vi "メイン.vi"() -> (2 "測定周期/ms":dbl, 3 "値転記用配列":T2[](array[typedef]))   [LabVIEW 2021] (continued)
                            n466 = Bundle By Name(cluster=w1247, "品質チェック項目"=w1249) -> (w1246:T2)
                          }
                          frame 7 {
                            n467 = call-poly <vilib>:"Read Key.vi"("section"=w1261, "error in (no error)"=w1260, "key"=w1257, "refnum"=w1263) -> ("error out"=w1259:errorcluster, "value"=w1258:i32, "refnum out"=w1262:T10)  [unwired: 4 in, 1 out]
                            n468 = Bundle By Name(cluster=w1256, "測定周期"=w1258) -> (w1255:T2)
                          }
                          frame 8 {
                            n469 = call-poly <vilib>:"Read Key.vi"("section"=w1270, "error in (no error)"=w1269, "key"=w1266, "refnum"=w1272) -> ("error out"=w1268:errorcluster, "value"=w1267:string, "refnum out"=w1271:T10)  [unwired: 4 in, 1 out]
                            n470 = Bundle By Name(cluster=w1264, "実測値MAX"=w1267) -> (w1265:T2)
                          }
                          frame 9 {
                            n471 = call-poly <vilib>:"Read Key.vi"("section"=w1279, "error in (no error)"=w1278, "key"=w1275, "refnum"=w1281) -> ("error out"=w1277:errorcluster, "value"=w1276:string, "refnum out"=w1280:T10)  [unwired: 4 in, 1 out]
                            n472 = Bundle By Name(cluster=w1273, "実測値MIN"=w1276) -> (w1274:T2)
                          }
                          frame 10 {
                            n473 = call-poly <vilib>:"Read Key.vi"("section"=w1288, "error in (no error)"=w1287, "key"=w1284, "refnum"=w1290) -> ("error out"=w1286:errorcluster, "value"=w1285:string, "refnum out"=w1289:T10)  [unwired: 4 in, 1 out]
                            n474 = Bundle By Name(cluster=w1282, "実測値(MAX)"=w1285) -> (w1283:T2)
                          }
                          frame 11 {
                            n475 = call-poly <vilib>:"Read Key.vi"("section"=w1297, "error in (no error)"=w1296, "key"=w1293, "refnum"=w1299) -> ("error out"=w1295:errorcluster, "value"=w1294:string, "refnum out"=w1298:T10)  [unwired: 4 in, 1 out]
                            n476 = Bundle By Name(cluster=w1291, "実測値(MIN)"=w1294) -> (w1292:T2)
                          }
                          frame 12 {
                            n477 = call-poly <vilib>:"Read Key.vi"("section"=w1306, "error in (no error)"=w1305, "key"=w1302, "refnum"=w1308) -> ("error out"=w1304:errorcluster, "value"=w1303:bool, "refnum out"=w1307:T10)  [unwired: 4 in, 1 out]
                            n478 = Bundle By Name(cluster=w1300, "測定画面表示ボタン"=w1303) -> (w1301:T2)
                          }
                          frame 13 {
                            n479 = call-poly <vilib>:"Read Key.vi"("section"=w1315, "error in (no error)"=w1314, "key"=w1311, "refnum"=w1317) -> ("error out"=w1313:errorcluster, "value"=w1312:string, "refnum out"=w1316:T10)  [unwired: 4 in, 1 out]
                            n480 = Bundle By Name(cluster=w1309, "ゲージポートNo"=w1312) -> (w1310:T2)
                          }
                        }
                        n481 = local write "メイン設定_設定 5"(w1185) -> ()
                      }
                      n482 = local read "メインON/OFF_\n設定 5"() -> (w1169:T1)
                      n483 = call-poly <vilib>:"Read Key.vi"("section"=w1158, "error in (no error)"=w1176, "key"="使用ON/OFF", "refnum"=w1177) -> ("error out"=w1161:errorcluster, "value"=w1167:bool, "refnum out"=w1162:T10)  [unwired: 4 in, 1 out]
                      n484 = Bundle By Name(cluster=w1169, "使用ON/OFF"=w1167) -> (w1170:T1)
                      n485 = local write "メインON/OFF_\n設定 5"(w1170) -> ()
                      n486 = local read "CSV項目名 5"() -> (w1165:T3)
                      n487 = call-poly <vilib>:"Read Key.vi"("section"=w1158, "error in (no error)"=w1161, "key"="CSVヘッダー名", "refnum"=w1162) -> ("error out"=w1159:errorcluster, "value"=w1163:string, "refnum out"=w1160:T10)  [unwired: 4 in, 1 out]
                      n488 = Bundle By Name(cluster=w1165, "CSV項目名"=w1163) -> (w1164:T3)
                      n489 = local write "CSV項目名 5"(w1164) -> ()
                    }
                    frame #1 {
                      # "csvヘッダー項目作成"
                      # "⑮"
                      # "⑤"
                      n490 = local read "CSV項目名 5"() -> (w1322:T3)
                      n491 = Unbundle By Name(w1322) -> ("CSV項目名"=w1319:string)
                      n492 = local read "メイン設定_設定 5"() -> (w1323:T2)
                      n493 = Unbundle By Name(w1323) -> ("測定モード"=w1318:u16)
                      n494 = case shown="0, デフォルト" w1318 {
                        tunnel: ["単発測定" _ "多点測定"] -> w1326
                        tunnel: [FALSE TRUE FALSE] -> w1325
                        tunnel: [TRUE FALSE TRUE] -> w1324
                        frame 0, Default {
                        }
                        frame 1 {
                        }
                        frame 2 {
                        }
                      }
                      n495 = case shown="1" w1318 {
                        tunnel: w1319 -> [w1332 w1344 w1353]
                        tunnel: [w1330 w1342 w1355] -> w1321
                        tunnel: [w1329 w1341 w1354] -> w1320
                        frame 1 {
                          n496 = Empty String/Path?(string/path=w1332) -> (empty?=w1331:bool)
                          n497 = case shown="FALSE" w1331 {
                            tunnel: w1332 -> [w1338 _]
                            tunnel: w1332 -> [w1337 _]
                            tunnel: [w1334 ""] -> w1330
                            tunnel: [w1333 ""] -> w1329
                            frame False {
                              n498 = Concatenate Strings(w1338, "_max") -> (w1334:string)
                              n499 = Concatenate Strings(w1337, "_min") -> (w1333:string)
                            }
                            frame True {
                            }
                          }
                        }
                        frame 2 {
                          n500 = Empty String/Path?(string/path=w1344) -> (empty?=w1343:bool)
                          n501 = case shown="FALSE" w1343 {
                            tunnel: w1344 -> [w1350 _]
                            tunnel: w1344 -> [w1349 _]
                            tunnel: [w1346 ""] -> w1342
                            tunnel: [w1345 ""] -> w1341
                            frame False {
                              n502 = Concatenate Strings(w1350, "_max") -> (w1346:string)
                              n503 = Concatenate Strings(w1349, "_min") -> (w1345:string)
                            }
                            frame True {
                            }
                          }
                        }
                        frame 0, Default {
                          n504 = Empty String/Path?(string/path=w1353) -> (empty?=w1356:bool)
                          n505 = case shown="FALSE" w1356 {
                            tunnel: w1353 -> [w1360 _]
                            tunnel: [w1358 ""] -> w1355
                            tunnel: ["" ""] -> w1354
                            frame False {
                              n506 = Concatenate Strings(w1360, "_value") -> (w1358:string)
                            }
                            frame True {
                            }
                          }
                        }
                      }
                      n507 = property on="メイン測定ボタン_単発 5" class="Bool (指定)"("BoolText.Text"=w1326) -> ()  [unwired: 2 in, 2 out]
                      n508 = local write "csv入力項目min 5"(w1320) -> ()
                      n509 = local write "csv入力項目max 5"(w1321) -> ()
                      n510 = property on="メイン測定ボタン_連続 5" class="Bool (指定)"("Visible"=w1325) -> ()  [unwired: 2 in, 2 out]
                      n511 = property on="メイン測定ボタン_単発 5" class="Bool (指定)"("Visible"=w1324) -> ()  [unwired: 2 in, 2 out]
                    }
                    frame #2 {
                      # "⑯"
                      # "⑨"
                      # "⑧"
                      # "⑦"
                      # "⑥"
                      n512 = local read "メインON/OFF_\n設定 5"() -> (w1374:T1)
                      n513 = local write "メインON/OFF_\n保存確認 5"(w1374) -> ()
                      n514 = local read "メイン設定_設定 5"() -> (w1372:T2)
                      n515 = Unbundle By Name(w1372) -> ("測定画面表示ボタン"=w1371:bool)
                      n516 = case shown="FALSE" w1371 {
                        tunnel: [w1377 TRUE] -> w1373
                        frame False {
                          w1377 = FALSE
                          n517 = property on="メイン測定ボタン_単発 5" class="Bool (指定)"("Visible"=w1377) -> ()  [unwired: 2 in, 2 out]
                          n518 = property on="メイン測定ボタン_連続 5" class="Bool (指定)"("Visible"=w1377) -> ()  [unwired: 2 in, 2 out]
                        }
                        frame True {
                        }
                      }
                      n519 = local write "メインON/OFF_制御器 5"(w1374) -> ()
                      n520 = property on="メインON/OFF_制御器 5" class="Clust (指定)"("Visible"=w1373) -> ()  [unwired: 2 in, 2 out]
                      n521 = property on="メイン設定No_設定 5" class="Clust (指定)"("Visible"=w1373) -> ()  [unwired: 2 in, 2 out]
                      n522 = property on="メイン設定_設定 5" class="Clust (指定)"("Visible"=w1373) -> ()  [unwired: 2 in, 2 out]
                      n523 = property on="キャンセルボタン 5" class="Bool (指定)"("Visible"=w1373) -> ()  [unwired: 2 in, 2 out]
                    }
                  }
                  n524 = Replace Array Subset(array=w1153, new element=w1146, index=4) -> (w1152:T2[])
                }
                frame 5 {
                  # "⑱"
                  # "⑰"
                  # "2つ目の配列に転記"
                  # "32回繰り返す為、増やす場合はこのケースストラクチャーを複製する\n複製時、設定項目の配列やボタンも複製する為、下記のボタン類の移動はしない事"
                  # "iniからデータ読み取り"
                  n525 = flat-sequence {
                    tunnel: w1388 -> [w1414]
                    tunnel: w1387 -> [w1415]
                    tunnel: [w1393] -> w1384
                    tunnel: [w1392] -> w1383
                    tunnel: w1384 -> [w1561]
                    tunnel: w1383 -> [w1560]
                    tunnel: [w1561] -> w1382
                    tunnel: [w1560] -> w1381
                    tunnel: [w1608] -> w1389
                    tunnel: [w1609] -> w1390
                    tunnel: w1382 -> [w1609]
                    tunnel: w1381 -> [w1608]
                    tunnel: [w1605] -> w1379
                    frame #0 {
                      w1391 = "設定6"
                      # "複製時に変更する項目\n①②③④⑤⑥⑦⑧⑨　⑪⑫\nローカル変数\n⑬⑭\nセレクション\n⑮⑯\nプロパティノードが\n対象配列になっているか確認\n⑰\n指標値\n⑱\n複製したケースのTrue定数を削除"
                      # "⑭"
                      # "⑬"
                      # "⑫"
                      # "⑪"
                      # "④"
                      # "③"
                      # "setting.iniファイルからの設定項目の読み取り"
                      n526 = local read "メイン設定No_設定 6"() -> (w1411:T5)
                      n527 = call-poly <vilib>:"Read Key.vi"("section"="No6.", "error in (no error)"=w1415, "key"="No.", "refnum"=w1414) -> ("error out"=w1408:errorcluster, "value"=w1412:i32, "refnum out"=w1406:T10)  [unwired: 4 in, 1 out]
                      n528 = Bundle By Name(cluster=w1411, "No."=w1412) -> (w1413:T5)
                      n529 = local write "メイン設定No_設定 6"(w1413) -> ()
                      n530 = for {
                        shift-right: [w1423] -> w1410
                        shift-left: w1406 -> [w1424]
                        shift-right: [w1420] -> w1409
                        shift-left: w1408 -> [w1421]
                        tunnel: string[] ["規格", "規格上限", "規格下限", "ポートNo.", "測定モード", "規格単位", "品質チェック項目", "測定周期", "実測MAX", "実測MIN", "実測(MAX)", "実測(MIN)", "測定画面表示ボタン", "ゲージポートNo."] -> [w1419] mode=indexing
                        tunnel: w1391 -> [w1416]
                        i -> [w1422]
                        # "②"
                        # "①"
                        n531 = local read "メイン設定_設定 6"() -> (w1417:T2)
                        n532 = case shown="0, デフォルト" w1422 {
                          tunnel: w1424 -> [w1433 w1442 w1451 w1460 w1469 w1478 w1487 w1496 w1505 w1514 w1523 w1532 w1541 w1550]
                          tunnel: [w1432 w1441 w1450 w1459 w1468 w1477 w1486 w1495 w1504 w1513 w1522 w1531 w1540 w1549] -> w1423
                          tunnel: w1416 -> [w1431 w1440 w1449 w1458 w1467 w1476 w1485 w1494 w1503 w1512 w1521 w1530 w1539 w1548]
                          tunnel: w1421 -> [w1430 w1439 w1448 w1457 w1466 w1475 w1484 w1493 w1502 w1511 w1520 w1529 w1538 w1547]
                          tunnel: [w1429 w1438 w1447 w1456 w1465 w1474 w1483 w1492 w1501 w1510 w1519 w1528 w1537 w1546] -> w1420
                          tunnel: w1419 -> [_ _ _ _ _ w1472 _ _ _ _ _ _ _ _]
                          tunnel: w1419 -> [_ _ _ _ _ _ w1481 _ _ _ _ w1526 _ _]
                          tunnel: w1419 -> [w1427 w1436 w1445 w1454 w1463 _ _ w1490 w1499 w1508 w1517 _ w1535 w1544]
                          tunnel: [w1426 w1435 w1444 w1453 w1462 w1470 w1479 w1488 w1498 w1507 w1516 w1525 w1534 w1543] -> w1418
                          tunnel: w1417 -> [w1425 w1434 w1443 w1452 w1461 w1471 w1480 w1489 w1497 w1506 w1515 w1524 w1533 w1542]
                          frame 0, Default {
                            n533 = call-poly <vilib>:"Read Key.vi"("section"=w1431, "error in (no error)"=w1430, "key"=w1427, "refnum"=w1433) -> ("error out"=w1429:errorcluster, "value"=w1428:string, "refnum out"=w1432:T10)  [unwired: 4 in, 1 out]
                            n534 = Bundle By Name(cluster=w1425, "規格"=w1428) -> (w1426:T2)
                          }
                          frame 1 {
                            n535 = call-poly <vilib>:"Read Key.vi"("section"=w1440, "error in (no error)"=w1439, "key"=w1436, "refnum"=w1442) -> ("error out"=w1438:errorcluster, "value"=w1437:string, "refnum out"=w1441:T10)  [unwired: 4 in, 1 out]
                            n536 = Bundle By Name(cluster=w1434, "規格上限"=w1437) -> (w1435:T2)
                          }
                          frame 2 {
                            n537 = call-poly <vilib>:"Read Key.vi"("section"=w1449, "error in (no error)"=w1448, "key"=w1445, "refnum"=w1451) -> ("error out"=w1447:errorcluster, "value"=w1446:string, "refnum out"=w1450:T10)  [unwired: 4 in, 1 out]
                            n538 = Bundle By Name(cluster=w1443, "規格下限"=w1446) -> (w1444:T2)
                          }
                          frame 3 {
                            n539 = call-poly <vilib>:"Read Key.vi"("section"=w1458, "error in (no error)"=w1457, "key"=w1454, "refnum"=w1460) -> ("error out"=w1456:errorcluster, "value"=w1455:i32, "refnum out"=w1459:T10)  [unwired: 4 in, 1 out]
                            n540 = Bundle By Name(cluster=w1452, "ポートNo."=w1455) -> (w1453:T2)
                          }
                          frame 4 {
                            n541 = call-poly <vilib>:"Read Key.vi"("section"=w1467, "error in (no error)"=w1466, "key"=w1463, "refnum"=w1469) -> ("error out"=w1465:errorcluster, "value"=w1464:i32, "refnum out"=w1468:T10)  [unwired: 4 in, 1 out]
                            n542 = Bundle By Name(cluster=w1461, "測定モード"=w1464) -> (w1462:T2)
                          }
                          frame 5 {
                            n543 = call-poly <vilib>:"Read Key.vi"("section"=w1476, "error in (no error)"=w1475, "key"=w1472, "refnum"=w1478) -> ("error out"=w1474:errorcluster, "value"=w1473:string, "refnum out"=w1477:T10)  [unwired: 4 in, 1 out]
                            n544 = Bundle By Name(cluster=w1471, "規格単位"=w1473) -> (w1470:T2)
                          }
                          frame 6 {
                            n545 = call-poly <vilib>:"Read Key.vi"("section"=w1485, "error in (no error)"=w1484, "key"=w1481, "refnum"=w1487) -> ("error out"=w1483:errorcluster, "value"=w1482:string, "refnum out"=w1486:T10)  [unwired: 4 in, 1 out]
                            n546 = Bundle By Name(cluster=w1480, "品質チェック項目"=w1482) -> (w1479:T2)
                          }
                          frame 7 {
                            n547 = call-poly <vilib>:"Read Key.vi"("section"=w1494, "error in (no error)"=w1493, "key"=w1490, "refnum"=w1496) -> ("error out"=w1492:errorcluster, "value"=w1491:i32, "refnum out"=w1495:T10)  [unwired: 4 in, 1 out]
                            n548 = Bundle By Name(cluster=w1489, "測定周期"=w1491) -> (w1488:T2)
                          }
                          frame 8 {
                            n549 = call-poly <vilib>:"Read Key.vi"("section"=w1503, "error in (no error)"=w1502, "key"=w1499, "refnum"=w1505) -> ("error out"=w1501:errorcluster, "value"=w1500:string, "refnum out"=w1504:T10)  [unwired: 4 in, 1 out]
                            n550 = Bundle By Name(cluster=w1497, "実測値MAX"=w1500) -> (w1498:T2)
                          }
                          frame 9 {
                            n551 = call-poly <vilib>:"Read Key.vi"("section"=w1512, "error in (no error)"=w1511, "key"=w1508, "refnum"=w1514) -> ("error out"=w1510:errorcluster, "value"=w1509:string, "refnum out"=w1513:T10)  [unwired: 4 in, 1 out]
                            n552 = Bundle By Name(cluster=w1506, "実測値MIN"=w1509) -> (w1507:T2)
                          }
                          frame 10 {
                            n553 = call-poly <vilib>:"Read Key.vi"("section"=w1521, "error in (no error)"=w1520, "key"=w1517, "refnum"=w1523) -> ("error out"=w1519:errorcluster, "value"=w1518:string, "refnum out"=w1522:T10)  [unwired: 4 in, 1 out]
                            n554 = Bundle By Name(cluster=w1515, "実測値(MAX)"=w1518) -> (w1516:T2)
                          }
                          frame 11 {
                            n555 = call-poly <vilib>:"Read Key.vi"("section"=w1530, "error in (no error)"=w1529, "key"=w1526, "refnum"=w1532) -> ("error out"=w1528:errorcluster, "value"=w1527:string, "refnum out"=w1531:T10)  [unwired: 4 in, 1 out]
                            n556 = Bundle By Name(cluster=w1524, "実測値(MIN)"=w1527) -> (w1525:T2)
                          }
                          frame 12 {
                            n557 = call-poly <vilib>:"Read Key.vi"("section"=w1539, "error in (no error)"=w1538, "key"=w1535, "refnum"=w1541) -> ("error out"=w1537:errorcluster, "value"=w1536:bool, "refnum out"=w1540:T10)  [unwired: 4 in, 1 out]
                            n558 = Bundle By Name(cluster=w1533, "測定画面表示ボタン"=w1536) -> (w1534:T2)
                          }
                          frame 13 {
                            n559 = call-poly <vilib>:"Read Key.vi"("section"=w1548, "error in (no error)"=w1547, "key"=w1544, "refnum"=w1550) -> ("error out"=w1546:errorcluster, "value"=w1545:string, "refnum out"=w1549:T10)  [unwired: 4 in, 1 out]
                            n560 = Bundle By Name(cluster=w1542, "ゲージポートNo"=w1545) -> (w1543:T2)
                          }
                        }
                        n561 = local write "メイン設定_設定 6"(w1418) -> ()
                      }
                      n562 = local read "メインON/OFF_\n設定 6"() -> (w1402:T1)
                      n563 = call-poly <vilib>:"Read Key.vi"("section"=w1391, "error in (no error)"=w1409, "key"="使用ON/OFF", "refnum"=w1410) -> ("error out"=w1394:errorcluster, "value"=w1400:bool, "refnum out"=w1395:T10)  [unwired: 4 in, 1 out]
                      n564 = Bundle By Name(cluster=w1402, "使用ON/OFF"=w1400) -> (w1403:T1)
                      n565 = local write "メインON/OFF_\n設定 6"(w1403) -> ()
                      n566 = local read "CSV項目名 6"() -> (w1398:T3)
                      n567 = call-poly <vilib>:"Read Key.vi"("section"=w1391, "error in (no error)"=w1394, "key"="CSVヘッダー名", "refnum"=w1395) -> ("error out"=w1392:errorcluster, "value"=w1396:string, "refnum out"=w1393:T10)  [unwired: 4 in, 1 out]
                      n568 = Bundle By Name(cluster=w1398, "CSV項目名"=w1396) -> (w1397:T3)
                      n569 = local write "CSV項目名 6"(w1397) -> ()
                    }
                    frame #1 {
                      # "csvヘッダー項目作成"
                      # "⑮"
                      # "⑤"
                      n570 = local read "CSV項目名 6"() -> (w1555:T3)
                      n571 = Unbundle By Name(w1555) -> ("CSV項目名"=w1552:string)
                      n572 = local read "メイン設定_設定 6"() -> (w1556:T2)
                      n573 = Unbundle By Name(w1556) -> ("測定モード"=w1551:u16)
                      n574 = case shown="0, デフォルト" w1551 {
                        tunnel: ["単発測定" _ "多点測定"] -> w1559
                        tunnel: [FALSE TRUE FALSE] -> w1558
                        tunnel: [TRUE FALSE TRUE] -> w1557
                        frame 0, Default {
                        }
                        frame 1 {
                        }
                        frame 2 {
                        }
                      }
                      n575 = case shown="1" w1551 {
                        tunnel: w1552 -> [w1565 w1577 w1586]
                        tunnel: [w1563 w1575 w1588] -> w1554
                        tunnel: [w1562 w1574 w1587] -> w1553
                        frame 1 {
                          n576 = Empty String/Path?(string/path=w1565) -> (empty?=w1564:bool)
                          n577 = case shown="FALSE" w1564 {
                            tunnel: w1565 -> [w1571 _]
                            tunnel: w1565 -> [w1570 _]
                            tunnel: [w1567 ""] -> w1563
                            tunnel: [w1566 ""] -> w1562
                            frame False {
                              n578 = Concatenate Strings(w1571, "_max") -> (w1567:string)
                              n579 = Concatenate Strings(w1570, "_min") -> (w1566:string)
                            }
                            frame True {
                            }
                          }
                        }
                        frame 2 {
                          n580 = Empty String/Path?(string/path=w1577) -> (empty?=w1576:bool)
                          n581 = case shown="FALSE" w1576 {
                            tunnel: w1577 -> [w1583 _]
                            tunnel: w1577 -> [w1582 _]
                            tunnel: [w1579 ""] -> w1575
                            tunnel: [w1578 ""] -> w1574
                            frame False {
                              n582 = Concatenate Strings(w1583, "_max") -> (w1579:string)
                              n583 = Concatenate Strings(w1582, "_min") -> (w1578:string)
                            }
                            frame True {
                            }
                          }
                        }
                        frame 0, Default {
                          n584 = Empty String/Path?(string/path=w1586) -> (empty?=w1589:bool)
                          n585 = case shown="FALSE" w1589 {
                            tunnel: w1586 -> [w1593 _]
                            tunnel: [w1591 ""] -> w1588
                            tunnel: ["" ""] -> w1587
                            frame False {
                              n586 = Concatenate Strings(w1593, "_value") -> (w1591:string)
                            }
                            frame True {
                            }
                          }
                        }
                      }
                      n587 = property on="メイン測定ボタン_単発 6" class="Bool (指定)"("BoolText.Text"=w1559) -> ()  [unwired: 2 in, 2 out]
                      n588 = local write "csv入力項目min 6"(w1553) -> ()
                      n589 = local write "csv入力項目max 6"(w1554) -> ()
                      n590 = property on="メイン測定ボタン_連続 6" class="Bool (指定)"("Visible"=w1558) -> ()  [unwired: 2 in, 2 out]
                      n591 = property on="メイン測定ボタン_単発 6" class="Bool (指定)"("Visible"=w1557) -> ()  [unwired: 2 in, 2 out]
                    }
                    frame #2 {
                      # "⑯"
                      # "⑨"
                      # "⑧"
                      # "⑦"
                      # "⑥"
                      n592 = local read "メインON/OFF_\n設定 6"() -> (w1607:T1)
                      n593 = local write "メインON/OFF_\n保存確認 6"(w1607) -> ()
                      n594 = local read "メイン設定_設定 6"() -> (w1605:T2)
                      n595 = Unbundle By Name(w1605) -> ("測定画面表示ボタン"=w1604:bool)
                      n596 = case shown="FALSE" w1604 {
                        tunnel: [w1610 TRUE] -> w1606
                        frame False {
                          w1610 = FALSE
                          n597 = property on="メイン測定ボタン_単発 6" class="Bool (指定)"("Visible"=w1610) -> ()  [unwired: 2 in, 2 out]
                          n598 = property on="メイン測定ボタン_連続 6" class="Bool (指定)"("Visible"=w1610) -> ()  [unwired: 2 in, 2 out]
                        }
                        frame True {
                        }
                      }
                      n599 = local write "メインON/OFF_制御器 6"(w1607) -> ()
                      n600 = property on="メインON/OFF_制御器 6" class="Clust (指定)"("Visible"=w1606) -> ()  [unwired: 2 in, 2 out]
                      n601 = property on="メイン設定No_設定 6" class="Clust (指定)"("Visible"=w1606) -> ()  [unwired: 2 in, 2 out]
                      n602 = property on="メイン設定_設定 6" class="Clust (指定)"("Visible"=w1606) -> ()  [unwired: 2 in, 2 out]
                      n603 = property on="キャンセルボタン 6" class="Bool (指定)"("Visible"=w1606) -> ()  [unwired: 2 in, 2 out]
                    }
                  }
                  n604 = Replace Array Subset(array=w1386, new element=w1379, index=5) -> (w1385:T2[])
                }
                frame 6 {
                  # "⑱"
                  # "⑰"
                  # "2つ目の配列に転記"
                  # "32回繰り返す為、増やす場合はこのケースストラクチャーを複製する\n複製時、設定項目の配列やボタンも複製する為、下記のボタン類の移動はしない事"
                  # "iniからデータ読み取り"
                  n605 = flat-sequence {
                    tunnel: w1621 -> [w1647]
                    tunnel: w1620 -> [w1648]
                    tunnel: [w1626] -> w1617
                    tunnel: [w1625] -> w1616
                    tunnel: w1617 -> [w1794]
                    tunnel: w1616 -> [w1793]
                    tunnel: [w1794] -> w1615
                    tunnel: [w1793] -> w1614
                    tunnel: [w1841] -> w1622
                    tunnel: [w1842] -> w1623
                    tunnel: w1615 -> [w1842]
                    tunnel: w1614 -> [w1841]
                    tunnel: [w1838] -> w1612
                    frame #0 {
                      w1624 = "設定7"
                      # "複製時に変更する項目\n①②③④⑤⑥⑦⑧⑨　⑪⑫\nローカル変数\n⑬⑭\nセレクション\n⑮⑯\nプロパティノードが\n対象配列になっているか確認\n⑰\n指標値\n⑱\n複製したケースのTrue定数を削除"
                      # "⑭"
                      # "⑬"
                      # "⑫"
                      # "⑪"
                      # "④"
                      # "③"
                      # "setting.iniファイルからの設定項目の読み取り"
                      n606 = local read "メイン設定No_設定 7"() -> (w1644:T5)
                      n607 = call-poly <vilib>:"Read Key.vi"("section"="No7.", "error in (no error)"=w1648, "key"="No.", "refnum"=w1647) -> ("error out"=w1641:errorcluster, "value"=w1645:i32, "refnum out"=w1639:T10)  [unwired: 4 in, 1 out]
                      n608 = Bundle By Name(cluster=w1644, "No."=w1645) -> (w1646:T5)
                      n609 = local write "メイン設定No_設定 7"(w1646) -> ()
                      n610 = for {
                        shift-right: [w1656] -> w1643
                        shift-left: w1639 -> [w1657]
                        shift-right: [w1653] -> w1642
                        shift-left: w1641 -> [w1654]
                        tunnel: string[] ["規格", "規格上限", "規格下限", "ポートNo.", "測定モード", "規格単位", "品質チェック項目", "測定周期", "実測MAX", "実測MIN", "実測(MAX)", "実測(MIN)", "測定画面表示ボタン", "ゲージポートNo."] -> [w1652] mode=indexing
                        tunnel: w1624 -> [w1649]
                        i -> [w1655]
                        # "②"
                        # "①"
                        n611 = local read "メイン設定_設定 7"() -> (w1650:T2)
                        n612 = case shown="0, デフォルト" w1655 {
                          tunnel: w1657 -> [w1666 w1675 w1684 w1693 w1702 w1711 w1720 w1729 w1738 w1747 w1756 w1765 w1774 w1783]
                          tunnel: [w1665 w1674 w1683 w1692 w1701 w1710 w1719 w1728 w1737 w1746 w1755 w1764 w1773 w1782] -> w1656
                          tunnel: w1649 -> [w1664 w1673 w1682 w1691 w1700 w1709 w1718 w1727 w1736 w1745 w1754 w1763 w1772 w1781]
                          tunnel: w1654 -> [w1663 w1672 w1681 w1690 w1699 w1708 w1717 w1726 w1735 w1744 w1753 w1762 w1771 w1780]
                          tunnel: [w1662 w1671 w1680 w1689 w1698 w1707 w1716 w1725 w1734 w1743 w1752 w1761 w1770 w1779] -> w1653
                          tunnel: w1652 -> [_ _ _ _ _ w1705 _ _ _ _ _ _ _ _]
                          tunnel: w1652 -> [_ _ _ _ _ _ w1714 _ _ _ _ w1759 _ _]
                          tunnel: w1652 -> [w1660 w1669 w1678 w1687 w1696 _ _ w1723 w1732 w1741 w1750 _ w1768 w1777]
                          tunnel: [w1659 w1668 w1677 w1686 w1695 w1703 w1712 w1721 w1731 w1740 w1749 w1758 w1767 w1776] -> w1651
                          tunnel: w1650 -> [w1658 w1667 w1676 w1685 w1694 w1704 w1713 w1722 w1730 w1739 w1748 w1757 w1766 w1775]
                          frame 0, Default {
                            n613 = call-poly <vilib>:"Read Key.vi"("section"=w1664, "error in (no error)"=w1663, "key"=w1660, "refnum"=w1666) -> ("error out"=w1662:errorcluster, "value"=w1661:string, "refnum out"=w1665:T10)  [unwired: 4 in, 1 out]
                            n614 = Bundle By Name(cluster=w1658, "規格"=w1661) -> (w1659:T2)
                          }
                          frame 1 {
                            n615 = call-poly <vilib>:"Read Key.vi"("section"=w1673, "error in (no error)"=w1672, "key"=w1669, "refnum"=w1675) -> ("error out"=w1671:errorcluster, "value"=w1670:string, "refnum out"=w1674:T10)  [unwired: 4 in, 1 out]
                            n616 = Bundle By Name(cluster=w1667, "規格上限"=w1670) -> (w1668:T2)
                          }
                          frame 2 {
                            n617 = call-poly <vilib>:"Read Key.vi"("section"=w1682, "error in (no error)"=w1681, "key"=w1678, "refnum"=w1684) -> ("error out"=w1680:errorcluster, "value"=w1679:string, "refnum out"=w1683:T10)  [unwired: 4 in, 1 out]
                            n618 = Bundle By Name(cluster=w1676, "規格下限"=w1679) -> (w1677:T2)
                          }
                          frame 3 {
                            n619 = call-poly <vilib>:"Read Key.vi"("section"=w1691, "error in (no error)"=w1690, "key"=w1687, "refnum"=w1693) -> ("error out"=w1689:errorcluster, "value"=w1688:i32, "refnum out"=w1692:T10)  [unwired: 4 in, 1 out]
                            n620 = Bundle By Name(cluster=w1685, "ポートNo."=w1688) -> (w1686:T2)
                          }
                          frame 4 {
                            n621 = call-poly <vilib>:"Read Key.vi"("section"=w1700, "error in (no error)"=w1699, "key"=w1696, "refnum"=w1702) -> ("error out"=w1698:errorcluster, "value"=w1697:i32, "refnum out"=w1701:T10)  [unwired: 4 in, 1 out]
                            n622 = Bundle By Name(cluster=w1694, "測定モード"=w1697) -> (w1695:T2)
                          }
                          frame 5 {
                            n623 = call-poly <vilib>:"Read Key.vi"("section"=w1709, "error in (no error)"=w1708, "key"=w1705, "refnum"=w1711) -> ("error out"=w1707:errorcluster, "value"=w1706:string, "refnum out"=w1710:T10)  [unwired: 4 in, 1 out]
                            n624 = Bundle By Name(cluster=w1704, "規格単位"=w1706) -> (w1703:T2)
                          }
                          frame 6 {
                            n625 = call-poly <vilib>:"Read Key.vi"("section"=w1718, "error in (no error)"=w1717, "key"=w1714, "refnum"=w1720) -> ("error out"=w1716:errorcluster, "value"=w1715:string, "refnum out"=w1719:T10)  [unwired: 4 in, 1 out]
                            n626 = Bundle By Name(cluster=w1713, "品質チェック項目"=w1715) -> (w1712:T2)
                          }
                          frame 7 {
                            n627 = call-poly <vilib>:"Read Key.vi"("section"=w1727, "error in (no error)"=w1726, "key"=w1723, "refnum"=w1729) -> ("error out"=w1725:errorcluster, "value"=w1724:i32, "refnum out"=w1728:T10)  [unwired: 4 in, 1 out]
                            n628 = Bundle By Name(cluster=w1722, "測定周期"=w1724) -> (w1721:T2)
                          }
                          frame 8 {
                            n629 = call-poly <vilib>:"Read Key.vi"("section"=w1736, "error in (no error)"=w1735, "key"=w1732, "refnum"=w1738) -> ("error out"=w1734:errorcluster, "value"=w1733:string, "refnum out"=w1737:T10)  [unwired: 4 in, 1 out]
                            n630 = Bundle By Name(cluster=w1730, "実測値MAX"=w1733) -> (w1731:T2)
                          }
                          frame 9 {
                            n631 = call-poly <vilib>:"Read Key.vi"("section"=w1745, "error in (no error)"=w1744, "key"=w1741, "refnum"=w1747) -> ("error out"=w1743:errorcluster, "value"=w1742:string, "refnum out"=w1746:T10)  [unwired: 4 in, 1 out]
                            n632 = Bundle By Name(cluster=w1739, "実測値MIN"=w1742) -> (w1740:T2)
                          }
                          frame 10 {
                            n633 = call-poly <vilib>:"Read Key.vi"("section"=w1754, "error in (no error)"=w1753, "key"=w1750, "refnum"=w1756) -> ("error out"=w1752:errorcluster, "value"=w1751:string, "refnum out"=w1755:T10)  [unwired: 4 in, 1 out]
                            n634 = Bundle By Name(cluster=w1748, "実測値(MAX)"=w1751) -> (w1749:T2)
                          }
                          frame 11 {
                            n635 = call-poly <vilib>:"Read Key.vi"("section"=w1763, "error in (no error)"=w1762, "key"=w1759, "refnum"=w1765) -> ("error out"=w1761:errorcluster, "value"=w1760:string, "refnum out"=w1764:T10)  [unwired: 4 in, 1 out]
                            n636 = Bundle By Name(cluster=w1757, "実測値(MIN)"=w1760) -> (w1758:T2)
                          }
                          frame 12 {
                            n637 = call-poly <vilib>:"Read Key.vi"("section"=w1772, "error in (no error)"=w1771, "key"=w1768, "refnum"=w1774) -> ("error out"=w1770:errorcluster, "value"=w1769:bool, "refnum out"=w1773:T10)  [unwired: 4 in, 1 out]
                            n638 = Bundle By Name(cluster=w1766, "測定画面表示ボタン"=w1769) -> (w1767:T2)
                          }
                          frame 13 {
                            n639 = call-poly <vilib>:"Read Key.vi"("section"=w1781, "error in (no error)"=w1780, "key"=w1777, "refnum"=w1783) -> ("error out"=w1779:errorcluster, "value"=w1778:string, "refnum out"=w1782:T10)  [unwired: 4 in, 1 out]
                            n640 = Bundle By Name(cluster=w1775, "ゲージポートNo"=w1778) -> (w1776:T2)
                          }
                        }
                        n641 = local write "メイン設定_設定 7"(w1651) -> ()
                      }
                      n642 = local read "メインON/OFF_\n設定 7"() -> (w1635:T1)
                      n643 = call-poly <vilib>:"Read Key.vi"("section"=w1624, "error in (no error)"=w1642, "key"="使用ON/OFF", "refnum"=w1643) -> ("error out"=w1627:errorcluster, "value"=w1633:bool, "refnum out"=w1628:T10)  [unwired: 4 in, 1 out]
                      n644 = Bundle By Name(cluster=w1635, "使用ON/OFF"=w1633) -> (w1636:T1)
                      n645 = local write "メインON/OFF_\n設定 7"(w1636) -> ()
                      n646 = local read "CSV項目名 7"() -> (w1631:T3)
                      n647 = call-poly <vilib>:"Read Key.vi"("section"=w1624, "error in (no error)"=w1627, "key"="CSVヘッダー名", "refnum"=w1628) -> ("error out"=w1625:errorcluster, "value"=w1629:string, "refnum out"=w1626:T10)  [unwired: 4 in, 1 out]
                      n648 = Bundle By Name(cluster=w1631, "CSV項目名"=w1629) -> (w1630:T3)
                      n649 = local write "CSV項目名 7"(w1630) -> ()
                    }
                    frame #1 {
                      # "csvヘッダー項目作成"
                      # "⑮"
                      # "⑤"
                      n650 = local read "CSV項目名 7"() -> (w1788:T3)
                      n651 = Unbundle By Name(w1788) -> ("CSV項目名"=w1785:string)
                      n652 = local read "メイン設定_設定 7"() -> (w1789:T2)
                      n653 = Unbundle By Name(w1789) -> ("測定モード"=w1784:u16)
                      n654 = case shown="0, デフォルト" w1784 {
                        tunnel: ["単発測定" _ "多点測定"] -> w1792
                        tunnel: [FALSE TRUE FALSE] -> w1791
                        tunnel: [TRUE FALSE TRUE] -> w1790
                        frame 0, Default {
                        }
                        frame 1 {
                        }
                        frame 2 {
                        }
                      }
                      n655 = case shown="1" w1784 {
                        tunnel: w1785 -> [w1798 w1810 w1819]
                        tunnel: [w1796 w1808 w1821] -> w1787
                        tunnel: [w1795 w1807 w1820] -> w1786
                        frame 1 {
                          n656 = Empty String/Path?(string/path=w1798) -> (empty?=w1797:bool)
                          n657 = case shown="FALSE" w1797 {
                            tunnel: w1798 -> [w1804 _]
                            tunnel: w1798 -> [w1803 _]
                            tunnel: [w1800 ""] -> w1796
                            tunnel: [w1799 ""] -> w1795
                            frame False {
                              n658 = Concatenate Strings(w1804, "_max") -> (w1800:string)
                              n659 = Concatenate Strings(w1803, "_min") -> (w1799:string)
                            }
                            frame True {
                            }
                          }
                        }
                        frame 2 {
                          n660 = Empty String/Path?(string/path=w1810) -> (empty?=w1809:bool)
                          n661 = case shown="FALSE" w1809 {
                            tunnel: w1810 -> [w1816 _]
                            tunnel: w1810 -> [w1815 _]
                            tunnel: [w1812 ""] -> w1808
                            tunnel: [w1811 ""] -> w1807
                            frame False {
                              n662 = Concatenate Strings(w1816, "_max") -> (w1812:string)
                              n663 = Concatenate Strings(w1815, "_min") -> (w1811:string)
                            }
                            frame True {
                            }
                          }
                        }
                        frame 0, Default {
                          n664 = Empty String/Path?(string/path=w1819) -> (empty?=w1822:bool)
                          n665 = case shown="FALSE" w1822 {
                            tunnel: w1819 -> [w1826 _]
                            tunnel: [w1824 ""] -> w1821
                            tunnel: ["" ""] -> w1820
                            frame False {
                              n666 = Concatenate Strings(w1826, "_value") -> (w1824:string)
                            }
                            frame True {
                            }
                          }
                        }
                      }
                      n667 = property on="メイン測定ボタン_単発 7" class="Bool (指定)"("BoolText.Text"=w1792) -> ()  [unwired: 2 in, 2 out]
                      n668 = local write "csv入力項目min 7"(w1786) -> ()
                      n669 = local write "csv入力項目max 7"(w1787) -> ()
                      n670 = property on="メイン測定ボタン_連続 7" class="Bool (指定)"("Visible"=w1791) -> ()  [unwired: 2 in, 2 out]
                      n671 = property on="メイン測定ボタン_単発 7" class="Bool (指定)"("Visible"=w1790) -> ()  [unwired: 2 in, 2 out]
                    }
                    frame #2 {
                      # "⑯"
                      # "⑨"
                      # "⑧"
                      # "⑦"
                      # "⑥"
                      n672 = local read "メインON/OFF_\n設定 7"() -> (w1840:T1)
                      n673 = local write "メインON/OFF_\n保存確認 7"(w1840) -> ()
                      n674 = local read "メイン設定_設定 7"() -> (w1838:T2)
                      n675 = Unbundle By Name(w1838) -> ("測定画面表示ボタン"=w1837:bool)
                      n676 = case shown="FALSE" w1837 {
                        tunnel: [w1843 TRUE] -> w1839
                        frame False {
                          w1843 = FALSE
                          n677 = property on="メイン測定ボタン_単発 7" class="Bool (指定)"("Visible"=w1843) -> ()  [unwired: 2 in, 2 out]
                          n678 = property on="メイン測定ボタン_連続 7" class="Bool (指定)"("Visible"=w1843) -> ()  [unwired: 2 in, 2 out]
                        }
                        frame True {
                        }
                      }
                      n679 = local write "メインON/OFF_制御器 7"(w1840) -> ()
                      n680 = property on="メインON/OFF_制御器 7" class="Clust (指定)"("Visible"=w1839) -> ()  [unwired: 2 in, 2 out]
                      n681 = property on="メイン設定No_設定 7" class="Clust (指定)"("Visible"=w1839) -> ()  [unwired: 2 in, 2 out]
                      n682 = property on="メイン設定_設定 7" class="Clust (指定)"("Visible"=w1839) -> ()  [unwired: 2 in, 2 out]
                      n683 = property on="キャンセルボタン 7" class="Bool (指定)"("Visible"=w1839) -> ()  [unwired: 2 in, 2 out]
                    }
                  }
                  n684 = Replace Array Subset(array=w1619, new element=w1612, index=6) -> (w1618:T2[])
                }
                frame 7 {
                  # "⑱"
                  # "⑰"
                  # "2つ目の配列に転記"
                  # "32回繰り返す為、増やす場合はこのケースストラクチャーを複製する\n複製時、設定項目の配列やボタンも複製する為、下記のボタン類の移動はしない事"
                  # "iniからデータ読み取り"
                  n685 = flat-sequence {
                    tunnel: w1854 -> [w1880]
                    tunnel: w1853 -> [w1881]
                    tunnel: [w1859] -> w1850
                    tunnel: [w1858] -> w1849
                    tunnel: w1850 -> [w2027]
                    tunnel: w1849 -> [w2026]
                    tunnel: [w2027] -> w1848
                    tunnel: [w2026] -> w1847
                    tunnel: [w2074] -> w1855
                    tunnel: [w2075] -> w1856
                    tunnel: w1848 -> [w2075]
                    tunnel: w1847 -> [w2074]
                    tunnel: [w2071] -> w1845
                    frame #0 {
                      w1857 = "設定8"
                      # "複製時に変更する項目\n①②③④⑤⑥⑦⑧⑨　⑪⑫\nローカル変数\n⑬⑭\nセレクション\n⑮⑯\nプロパティノードが\n対象配列になっているか確認\n⑰\n指標値\n⑱\n複製したケースのTrue定数を削除"
                      # "⑭"
                      # "⑬"
                      # "⑫"
                      # "⑪"
                      # "④"
                      # "③"
                      # "setting.iniファイルからの設定項目の読み取り"
                      n686 = local read "メイン設定No_設定 8"() -> (w1877:T5)
                      n687 = call-poly <vilib>:"Read Key.vi"("section"="No8.", "error in (no error)"=w1881, "key"="No.", "refnum"=w1880) -> ("error out"=w1874:errorcluster, "value"=w1878:i32, "refnum out"=w1872:T10)  [unwired: 4 in, 1 out]
                      n688 = Bundle By Name(cluster=w1877, "No."=w1878) -> (w1879:T5)
                      n689 = local write "メイン設定No_設定 8"(w1879) -> ()
                      n690 = for {
                        shift-right: [w1889] -> w1876
                        shift-left: w1872 -> [w1890]
                        shift-right: [w1886] -> w1875
                        shift-left: w1874 -> [w1887]
                        tunnel: string[] ["規格", "規格上限", "規格下限", "ポートNo.", "測定モード", "規格単位", "品質チェック項目", "測定周期", "実測MAX", "実測MIN", "実測(MAX)", "実測(MIN)", "測定画面表示ボタン", "ゲージポートNo."] -> [w1885] mode=indexing
                        tunnel: w1857 -> [w1882]
                        i -> [w1888]
                        # "②"
                        # "①"
                        n691 = local read "メイン設定_設定 8"() -> (w1883:T2)
                        n692 = case shown="0, デフォルト" w1888 {
                          tunnel: w1890 -> [w1899 w1908 w1917 w1926 w1935 w1944 w1953 w1962 w1971 w1980 w1989 w1998 w2007 w2016]
                          tunnel: [w1898 w1907 w1916 w1925 w1934 w1943 w1952 w1961 w1970 w1979 w1988 w1997 w2006 w2015] -> w1889
                          tunnel: w1882 -> [w1897 w1906 w1915 w1924 w1933 w1942 w1951 w1960 w1969 w1978 w1987 w1996 w2005 w2014]
                          tunnel: w1887 -> [w1896 w1905 w1914 w1923 w1932 w1941 w1950 w1959 w1968 w1977 w1986 w1995 w2004 w2013]
                          tunnel: [w1895 w1904 w1913 w1922 w1931 w1940 w1949 w1958 w1967 w1976 w1985 w1994 w2003 w2012] -> w1886
                          tunnel: w1885 -> [_ _ _ _ _ w1938 _ _ _ _ _ _ _ _]
                          tunnel: w1885 -> [_ _ _ _ _ _ w1947 _ _ _ _ w1992 _ _]
                          tunnel: w1885 -> [w1893 w1902 w1911 w1920 w1929 _ _ w1956 w1965 w1974 w1983 _ w2001 w2010]
                          tunnel: [w1892 w1901 w1910 w1919 w1928 w1936 w1945 w1954 w1964 w1973 w1982 w1991 w2000 w2009] -> w1884
                          tunnel: w1883 -> [w1891 w1900 w1909 w1918 w1927 w1937 w1946 w1955 w1963 w1972 w1981 w1990 w1999 w2008]
                          frame 0, Default {
                            n693 = call-poly <vilib>:"Read Key.vi"("section"=w1897, "error in (no error)"=w1896, "key"=w1893, "refnum"=w1899) -> ("error out"=w1895:errorcluster, "value"=w1894:string, "refnum out"=w1898:T10)  [unwired: 4 in, 1 out]
                            n694 = Bundle By Name(cluster=w1891, "規格"=w1894) -> (w1892:T2)
                          }
                          frame 1 {
                            n695 = call-poly <vilib>:"Read Key.vi"("section"=w1906, "error in (no error)"=w1905, "key"=w1902, "refnum"=w1908) -> ("error out"=w1904:errorcluster, "value"=w1903:string, "refnum out"=w1907:T10)  [unwired: 4 in, 1 out]
                            n696 = Bundle By Name(cluster=w1900, "規格上限"=w1903) -> (w1901:T2)
                          }
                          frame 2 {
                            n697 = call-poly <vilib>:"Read Key.vi"("section"=w1915, "error in (no error)"=w1914, "key"=w1911, "refnum"=w1917) -> ("error out"=w1913:errorcluster, "value"=w1912:string, "refnum out"=w1916:T10)  [unwired: 4 in, 1 out]
                            n698 = Bundle By Name(cluster=w1909, "規格下限"=w1912) -> (w1910:T2)
                          }
                          frame 3 {
                            n699 = call-poly <vilib>:"Read Key.vi"("section"=w1924, "error in (no error)"=w1923, "key"=w1920, "refnum"=w1926) -> ("error out"=w1922:errorcluster, "value"=w1921:i32, "refnum out"=w1925:T10)  [unwired: 4 in, 1 out]
                            n700 = Bundle By Name(cluster=w1918, "ポートNo."=w1921) -> (w1919:T2)
                          }
                          frame 4 {
                            n701 = call-poly <vilib>:"Read Key.vi"("section"=w1933, "error in (no error)"=w1932, "key"=w1929, "refnum"=w1935) -> ("error out"=w1931:errorcluster, "value"=w1930:i32, "refnum out"=w1934:T10)  [unwired: 4 in, 1 out]
                            n702 = Bundle By Name(cluster=w1927, "測定モード"=w1930) -> (w1928:T2)
                          }
                          frame 5 {
                            n703 = call-poly <vilib>:"Read Key.vi"("section"=w1942, "error in (no error)"=w1941, "key"=w1938, "refnum"=w1944) -> ("error out"=w1940:errorcluster, "value"=w1939:string, "refnum out"=w1943:T10)  [unwired: 4 in, 1 out]
                            n704 = Bundle By Name(cluster=w1937, "規格単位"=w1939) -> (w1936:T2)
                          }
                          frame 6 {
                            n705 = call-poly <vilib>:"Read Key.vi"("section"=w1951, "error in (no error)"=w1950, "key"=w1947, "refnum"=w1953) -> ("error out"=w1949:errorcluster, "value"=w1948:string, "refnum out"=w1952:T10)  [unwired: 4 in, 1 out]
                            n706 = Bundle By Name(cluster=w1946, "品質チェック項目"=w1948) -> (w1945:T2)
                          }
                          frame 7 {
                            n707 = call-poly <vilib>:"Read Key.vi"("section"=w1960, "error in (no error)"=w1959, "key"=w1956, "refnum"=w1962) -> ("error out"=w1958:errorcluster, "value"=w1957:i32, "refnum out"=w1961:T10)  [unwired: 4 in, 1 out]
                            n708 = Bundle By Name(cluster=w1955, "測定周期"=w1957) -> (w1954:T2)
                          }
                          frame 8 {
                            n709 = call-poly <vilib>:"Read Key.vi"("section"=w1969, "error in (no error)"=w1968, "key"=w1965, "refnum"=w1971) -> ("error out"=w1967:errorcluster, "value"=w1966:string, "refnum out"=w1970:T10)  [unwired: 4 in, 1 out]
                            n710 = Bundle By Name(cluster=w1963, "実測値MAX"=w1966) -> (w1964:T2)
                          }
                          frame 9 {
                            n711 = call-poly <vilib>:"Read Key.vi"("section"=w1978, "error in (no error)"=w1977, "key"=w1974, "refnum"=w1980) -> ("error out"=w1976:errorcluster, "value"=w1975:string, "refnum out"=w1979:T10)  [unwired: 4 in, 1 out]
                            n712 = Bundle By Name(cluster=w1972, "実測値MIN"=w1975) -> (w1973:T2)
                          }
                          frame 10 {
                            n713 = call-poly <vilib>:"Read Key.vi"("section"=w1987, "error in (no error)"=w1986, "key"=w1983, "refnum"=w1989) -> ("error out"=w1985:errorcluster, "value"=w1984:string, "refnum out"=w1988:T10)  [unwired: 4 in, 1 out]
                            n714 = Bundle By Name(cluster=w1981, "実測値(MAX)"=w1984) -> (w1982:T2)
                          }
                          frame 11 {
                            n715 = call-poly <vilib>:"Read Key.vi"("section"=w1996, "error in (no error)"=w1995, "key"=w1992, "refnum"=w1998) -> ("error out"=w1994:errorcluster, "value"=w1993:string, "refnum out"=w1997:T10)  [unwired: 4 in, 1 out]
                            n716 = Bundle By Name(cluster=w1990, "実測値(MIN)"=w1993) -> (w1991:T2)
                          }
                          frame 12 {
                            n717 = call-poly <vilib>:"Read Key.vi"("section"=w2005, "error in (no error)"=w2004, "key"=w2001, "refnum"=w2007) -> ("error out"=w2003:errorcluster, "value"=w2002:bool, "refnum out"=w2006:T10)  [unwired: 4 in, 1 out]
                            n718 = Bundle By Name(cluster=w1999, "測定画面表示ボタン"=w2002) -> (w2000:T2)
                          }
                          frame 13 {
                            n719 = call-poly <vilib>:"Read Key.vi"("section"=w2014, "error in (no error)"=w2013, "key"=w2010, "refnum"=w2016) -> ("error out"=w2012:errorcluster, "value"=w2011:string, "refnum out"=w2015:T10)  [unwired: 4 in, 1 out]
                            n720 = Bundle By Name(cluster=w2008, "ゲージポートNo"=w2011) -> (w2009:T2)
                          }
                        }
                        n721 = local write "メイン設定_設定 8"(w1884) -> ()
                      }
                      n722 = local read "メインON/OFF_\n設定 8"() -> (w1868:T1)
                      n723 = call-poly <vilib>:"Read Key.vi"("section"=w1857, "error in (no error)"=w1875, "key"="使用ON/OFF", "refnum"=w1876) -> ("error out"=w1860:errorcluster, "value"=w1866:bool, "refnum out"=w1861:T10)  [unwired: 4 in, 1 out]
                      n724 = Bundle By Name(cluster=w1868, "使用ON/OFF"=w1866) -> (w1869:T1)
                      n725 = local write "メインON/OFF_\n設定 8"(w1869) -> ()
                      n726 = local read "CSV項目名 8"() -> (w1864:T3)
                      n727 = call-poly <vilib>:"Read Key.vi"("section"=w1857, "error in (no error)"=w1860, "key"="CSVヘッダー名", "refnum"=w1861) -> ("error out"=w1858:errorcluster, "value"=w1862:string, "refnum out"=w1859:T10)  [unwired: 4 in, 1 out]
                      n728 = Bundle By Name(cluster=w1864, "CSV項目名"=w1862) -> (w1863:T3)
                      n729 = local write "CSV項目名 8"(w1863) -> ()
                    }
                    frame #1 {
                      # "csvヘッダー項目作成"
                      # "⑮"
                      # "⑤"
                      n730 = local read "CSV項目名 8"() -> (w2021:T3)
                      n731 = Unbundle By Name(w2021) -> ("CSV項目名"=w2018:string)
                      n732 = local read "メイン設定_設定 8"() -> (w2022:T2)
                      n733 = Unbundle By Name(w2022) -> ("測定モード"=w2017:u16)
                      n734 = case shown="0, デフォルト" w2017 {
                        tunnel: ["単発測定" _ "多点測定"] -> w2025
                        tunnel: [FALSE TRUE FALSE] -> w2024
                        tunnel: [TRUE FALSE TRUE] -> w2023
                        frame 0, Default {
                        }
                        frame 1 {
                        }
                        frame 2 {
                        }
                      }
                      n735 = case shown="1" w2017 {
                        tunnel: w2018 -> [w2031 w2043 w2052]
                        tunnel: [w2029 w2041 w2054] -> w2020
                        tunnel: [w2028 w2040 w2053] -> w2019
                        frame 1 {
                          n736 = Empty String/Path?(string/path=w2031) -> (empty?=w2030:bool)
                          n737 = case shown="FALSE" w2030 {
                            tunnel: w2031 -> [w2037 _]
                            tunnel: w2031 -> [w2036 _]
                            tunnel: [w2033 ""] -> w2029
                            tunnel: [w2032 ""] -> w2028
                            frame False {
                              n738 = Concatenate Strings(w2037, "_max") -> (w2033:string)
                              n739 = Concatenate Strings(w2036, "_min") -> (w2032:string)
                            }
                            frame True {
                            }
                          }
                        }
                        frame 2 {
                          n740 = Empty String/Path?(string/path=w2043) -> (empty?=w2042:bool)
                          n741 = case shown="FALSE" w2042 {
                            tunnel: w2043 -> [w2049 _]
                            tunnel: w2043 -> [w2048 _]
                            tunnel: [w2045 ""] -> w2041
                            tunnel: [w2044 ""] -> w2040
                            frame False {
                              n742 = Concatenate Strings(w2049, "_max") -> (w2045:string)
                              n743 = Concatenate Strings(w2048, "_min") -> (w2044:string)
                            }
                            frame True {
                            }
                          }
                        }
                        frame 0, Default {
                          n744 = Empty String/Path?(string/path=w2052) -> (empty?=w2055:bool)
                          n745 = case shown="FALSE" w2055 {
                            tunnel: w2052 -> [w2059 _]
                            tunnel: [w2057 ""] -> w2054
                            tunnel: ["" ""] -> w2053
                            frame False {
                              n746 = Concatenate Strings(w2059, "_value") -> (w2057:string)
                            }
                            frame True {
                            }
                          }
                        }
                      }
